vi "Save-As-Default (SubVI).vi"(0 "Current VI's Path":path, 1 "Load Settings":bool, 9 "Save Settings":bool, 12 "Save and Exit":bool) -> (4 "appended path":path, 8 "Save as Default Error":errorcluster, 15 "Application:Kind":T1(ring))   [LabVIEW 2012]
panel:
  # "Save As Defaults (SubVI) - Created by Blake Otting - October 2007"
  # "Last Updated 7/21/09"
  # "Connect As Shown \nin Main Program VI"
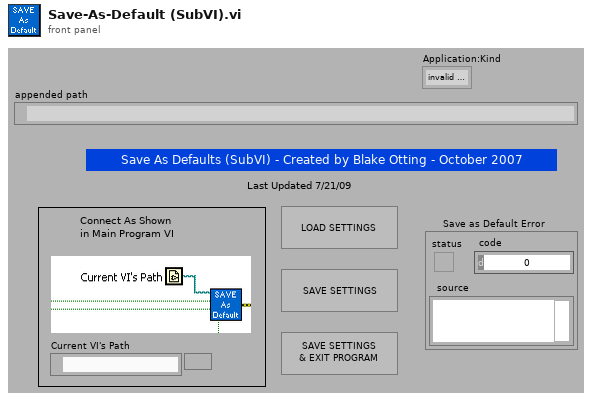
[diagram p1: front panel]
types:
  T1 = enum32{"invalid app kind", "Development System", "Run Time System", "Student Edition", "Embedded LabVIEW", "Evaluation", "Custom"}
  T2 = enum16{"open", "replace", "create", "open or create", "replace or create", "replace or create with confirmation"}
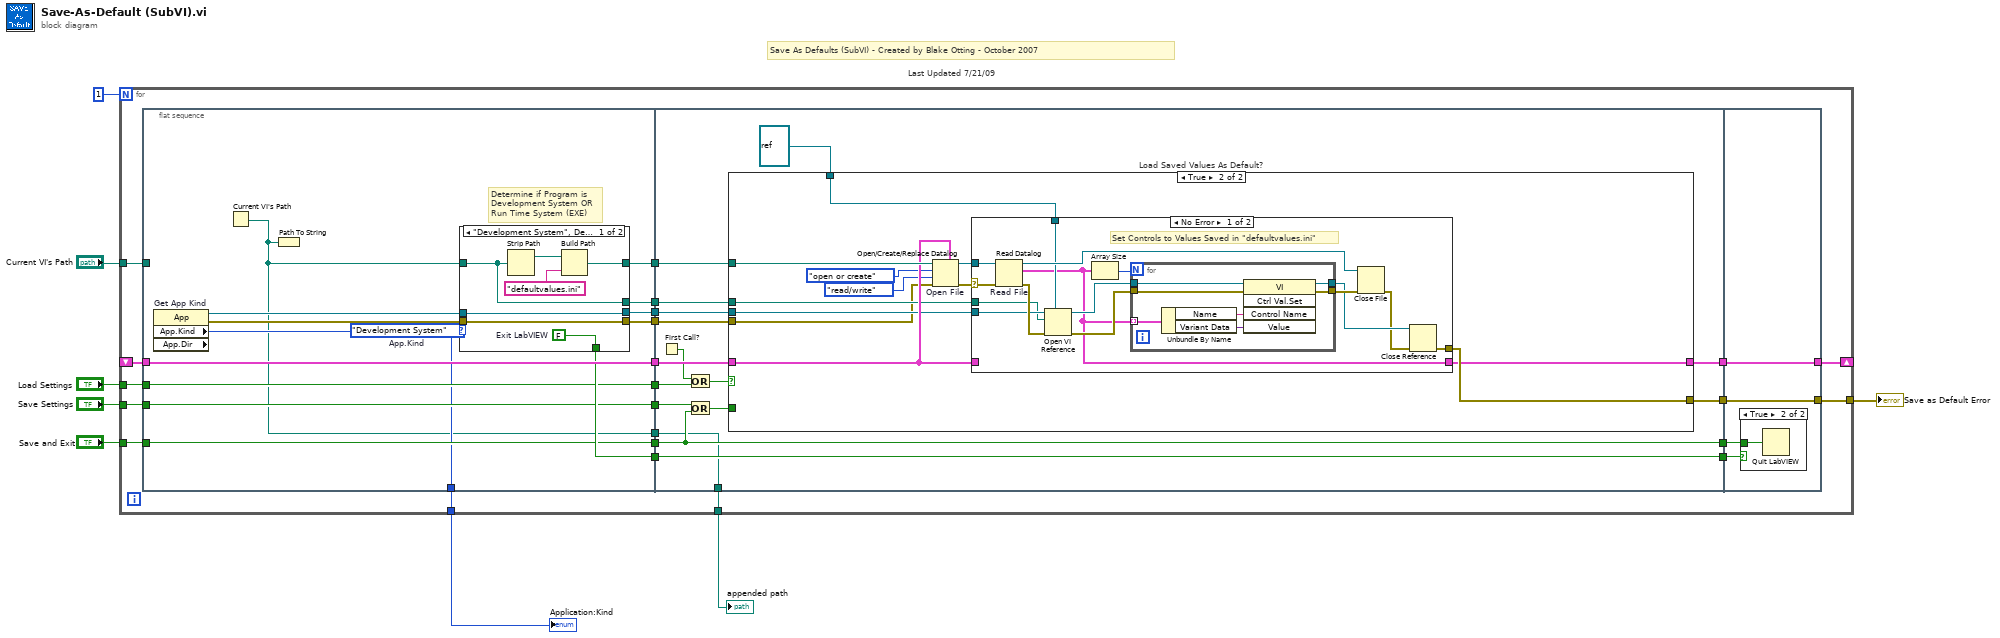
[diagram p0: block diagram]
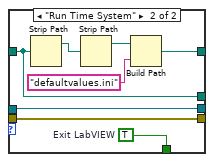
[diagram p2: hidden frame]
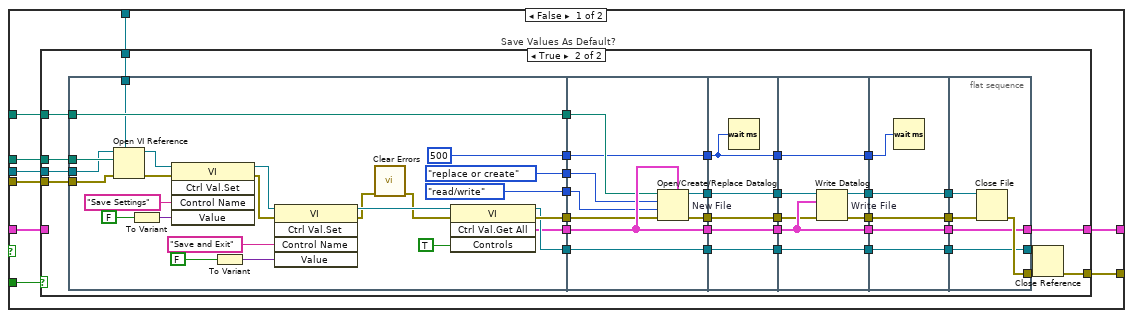
[diagram p3: hidden frame]
diagram:
  # "Last Updated 7/21/09"
  # "Save As Defaults (SubVI) - Created by Blake Otting - October 2007"
  n1 = for {
    N: 1 -> [_]
    tunnel: "Current VI's Path" -> [w30]
    shift-right: [w31] -> _
    shift-left: _ -> [w29]
    tunnel: [w28] -> w3
    tunnel: "Save and Exit" -> [w14]
    tunnel: "Load Settings" -> [w12]
    tunnel: "Save Settings" -> [w16]
    tunnel: [w11] -> w2
    tunnel: [w10] -> w1
    n2 = flat-sequence {
      tunnel: w30 -> [_]
      tunnel: w29 -> [w45]
      tunnel: [w45] -> w24
      tunnel: [w42] -> w23
      tunnel: [w41] -> w22
      tunnel: [w40] -> w21
      tunnel: [w39] -> w20
      tunnel: [w38] -> w19
      tunnel: [w37] -> w17
      tunnel: w16 -> [w37]
      tunnel: [w36] -> w15
      tunnel: w14 -> [w36]
      tunnel: [w35] -> w13
      tunnel: w12 -> [w35]
      tunnel: [w34] -> w11
      tunnel: [w32] -> w9
      tunnel: [w75] -> w27
      tunnel: [w68] -> w26
      tunnel: [w71] -> w25
      tunnel: w24 -> [w76]
      tunnel: w23 -> [w61]
      tunnel: w22 -> [w69]
      tunnel: w21 -> [w68]
      tunnel: w20 -> [w67]
      tunnel: w19 -> [w66]
      tunnel: [w65] -> w18
      tunnel: w17 -> [w64]
      tunnel: w15 -> [w65]
      tunnel: w13 -> [w63]
      tunnel: [w62] -> w10
      tunnel: w9 -> [w62]
      tunnel: [w217] -> w28
      tunnel: [w218] -> w31
      tunnel: w27 -> [w218]
      tunnel: w26 -> [w216]
      tunnel: w25 -> [w217]
      tunnel: w18 -> [w215]
      frame #0 {
        w33 = T1."Development System"  # App.Kind
        # "Determine if Program is\nDevelopment System OR\nRun Time System (EXE)"
        n3 = property on="Get App Kind" class="App" props=["App.Kind", "App.Dir"]() -> (reference out=w44:refnum<vi>, error out=w43:errorcluster, "App.Kind"=w34:T1)  [unwired: 2 in, 1 out]
        n4 = Current VI's Path() -> (path=w32:path)
        n5 = Path To String(path=w32) -> ()  [unwired: 1 out]
        n6 = case shown="\"Development System\", Default" w33 {
          tunnel: w43 -> [w52 w60]
          tunnel: [w52 w60] -> w41
          tunnel: w32 -> [w47 w54]
          tunnel: [w50 w56] -> w42
          tunnel: w44 -> [w48 w55]
          tunnel: [w48 w55] -> w38
          tunnel: [w47 w54] -> w39
          tunnel: [w46 w53] -> w40
          frame "Development System", Default {
            w46 = FALSE  # Exit LabVIEW
            n7 = Strip Path(path=w47) -> (stripped path=w49:path)  [unwired: 1 out]
            n8 = Build Path(base path=w49, name or relative path="defaultvalues.ini") -> (appended path=w50:path)
          }
          frame "Run Time System" {
            w53 = TRUE  # Exit LabVIEW
            n9 = Strip Path(path=w54) -> (stripped path=w57:path)  [unwired: 1 out]
            n10 = Strip Path(path=w57) -> (stripped path=w59:path)  [unwired: 1 out]
            n11 = Build Path(base path=w59, name or relative path="defaultvalues.ini") -> (appended path=w56:path)
          }
        }
      }
      frame #1 {
        n12 = First Call?() -> (First Call?: T/F=w70:bool)
        n13 = Or(x=w70, y=w63) -> (x .or. y?=w73:bool)
        n14 = Or(x=w64, y=w65) -> (x .or. y?=w72:bool)
        n15 = case "Load Saved Values As Default?" shown="True" w73 {
          tunnel: w69 -> [w85 w183]
          tunnel: [w84 w190] -> w71
          tunnel: w61 -> [w83 w188]
          tunnel: w72 -> [w82 _]
          tunnel: w76 -> [w81 w187]
          tunnel: [w77 w189] -> w75
          tunnel: w67 -> [w80 w184]
          tunnel: w66 -> [w79 w186]
          tunnel: refnum<vi> refnum ("Application Reference Input 2") -> [w78 w185]
          frame False {
            n16 = case "Save Values As Default?" shown="True" w82 {
              tunnel: w85 -> [w87 w88]
              tunnel: [w87 w122] -> w84
              tunnel: w83 -> [_ w121]
              tunnel: [w86 w120] -> w77
              tunnel: w81 -> [w86 _]
              tunnel: w80 -> [_ w90]
              tunnel: w79 -> [_ w89]
              tunnel: w78 -> [_ w91]
              frame False {
              }
              frame True {
                n17 = flat-sequence {
                  tunnel: w121 -> [w147]
                  tunnel: [w128] -> w100
                  tunnel: [enum16{"read/write", "read-only", "write-only"}."read/write" ("access (0:read/write)")] -> w99
                  tunnel: [T2."replace or create" ("operation (0:open)")] -> w98
                  tunnel: [w126] -> w97
                  tunnel: [w147] -> w96
                  tunnel: [w127] -> w95
                  tunnel: [u32 500 ("milliseconds to wait")] -> w94
                  tunnel: w91 -> [w131]
                  tunnel: w90 -> [w130]
                  tunnel: w89 -> [w129]
                  tunnel: w88 -> [w125]
                  tunnel: [w152] -> w119
                  tunnel: [w151] -> w117
                  tunnel: [w156] -> w115
                  tunnel: [w149] -> w113
                  tunnel: [w148] -> w101
                  tunnel: w100 -> [w155]
                  tunnel: w99 -> [w154]
                  tunnel: w98 -> [w153]
                  tunnel: w97 -> [w156]
                  tunnel: w96 -> [w150]
                  tunnel: w95 -> [w149]
                  tunnel: w94 -> [w148]
                  tunnel: w119 -> [w161]
                  tunnel: [w161] -> w118
                  tunnel: w117 -> [w160]
                  tunnel: [w160] -> w116
                  tunnel: w115 -> [w159]
                  tunnel: [w159] -> w114
                  tunnel: w113 -> [w158]
                  tunnel: [w158] -> w112
                  tunnel: w101 -> [w157]
                  tunnel: [w157] -> w92
                  tunnel: w118 -> [w166]
                  tunnel: w116 -> [w168]
                  tunnel: w114 -> [w167]
                  tunnel: [w167] -> w111
                  tunnel: w112 -> [w165]
                  tunnel: [w165] -> w109
                  tunnel: [w164] -> w107
                  tunnel: [w163] -> w105
                  tunnel: [w162] -> w93
                  tunnel: w92 -> [w162]
                  tunnel: w111 -> [w173]
                  tunnel: [w173] -> w110
                  tunnel: w109 -> [w172]
                  tunnel: [w172] -> w108
                  tunnel: w107 -> [w171]
                  tunnel: [w171] -> w106
                  tunnel: w105 -> [w170]
                  tunnel: [w170] -> w104
                  tunnel: w93 -> [w169]
                  tunnel: [w177] -> w120
                  tunnel: w110 -> [w177]
                  tunnel: [w176] -> w102
                  tunnel: w108 -> [w176]
                  tunnel: w106 -> [w175]
                  tunnel: w104 -> [w174]
                  tunnel: [w178] -> w103
                  frame #0 {
                    n18 = Open VI Reference(type specifier VI Refnum (for type only)=w131, application reference (local)=w129, vi path=w130, error in (no error)=w125) -> (vi reference=w139:refnum<vi>, error out=w140:errorcluster)  [unwired: 2 out]
                    n19 = To Variant(anything=FALSE ("Controls")) -> (Variant=w138:variant)
                    n20 = invoke class="VI" method="Ctrl Val.Set"(reference=w139, error in=w140, "Control Name"="Save Settings", "Value"=w138) -> (reference out=w143:refnum<vi>, error out=w144:errorcluster)  [unwired: 1 in, 3 out]
                    n21 = To Variant(anything=FALSE ("Controls")) -> (Variant=w141:variant)
                    n22 = invoke class="VI" method="Ctrl Val.Set"(reference=w143, error in=w144, "Control Name"="Save and Exit", "Value"=w141) -> (reference out=w146:refnum<vi>, error out=w124:errorcluster)  [unwired: 1 in, 3 out]
                    n23 = call <vilib>:"Clear Errors.vi"("error in (no error)"=w124) -> ("error out"=w123:errorcluster)  [unwired: 6 out]
                    n24 = invoke class="VI" method="Ctrl Val.Get All"(reference=w146, error in=w123, "Controls"=TRUE) -> (reference out=w127:refnum<vi>, error out=w128:errorcluster, "Get All Control Values Variant"=w126:cluster{"Name":string, "Variant Data":variant}[])  [unwired: 1 in, 1 out]
                  }
                  frame #1 {
                    n25 = Open/Create/Replace Datalog "New File"(5:w156, 8:w155, 9:w154, 10:w153, 11:w150) -> (0:w152:errorcluster, 3:w151:refnum<k1>)  [unwired: 2 out]
                  }
                  frame #2 {
                    n26 = Wait (ms)(milliseconds to wait=w157) -> ()  [unwired: 1 out]
                  }
                  frame #3 {
                    n27 = Write Datalog "Write File"(4:w166, 6:w167, 7:w168) -> (0:w164:errorcluster, 3:w163:refnum<k1>)
                  }
                  frame #4 {
                    n28 = Wait (ms)(milliseconds to wait=w169) -> ()  [unwired: 1 out]
                  }
                  frame #5 {
                    n29 = Close File(refnum=w174, error in=w175) -> (error out=w178:errorcluster)  [unwired: 1 out]
                  }
                }
                n30 = Close Reference(reference=w102, error in (no error)=w103) -> (error out=w122:errorcluster)
              }
            }
          }
          frame True {
            n31 = Open/Create/Replace Datalog "Open File"(5:w187, 8:w183, 9:enum16{"read/write", "read-only", "write-only"}."read/write" ("access (0:read/write)"), 10:T2."open or create" ("operation (0:open)"), 11:w188) -> (0:w182:errorcluster, 3:w181:refnum<k1>)  [unwired: 2 out]
            n32 = case shown="No Error" w182 {
              selector: w182 -> [w199 w213]
              tunnel: [w203 w213] -> w190
              tunnel: w187 -> [_ w214]
              tunnel: [w191 w214] -> w189
              tunnel: w181 -> [w200 _]
              tunnel: w186 -> [w196 _]
              tunnel: w185 -> [w195 _]
              tunnel: w184 -> [w194 _]
              frame No Error {
                # "Set Controls to Values Saved in \"defaultvalues.ini\""
                n33 = Read Datalog "Read File"(4:w199, 7:w200) -> (0:w197:errorcluster, 2:w191:cluster{"Name":string, "Variant Data":variant}[], 3:w205:refnum<k1>)  [unwired: 1 out]
                n34 = Open VI Reference(type specifier VI Refnum (for type only)=w195, application reference (local)=w196, vi path=w194, error in (no error)=w197) -> (vi reference=w198:refnum<vi>, error out=w193:errorcluster)  [unwired: 2 out]
                n35 = Array Size(array=w191) -> (size(s)=w192:i32)
                n36 = for {
                  N: w192 -> [_]
                  tunnel: w191 -> [w208] mode=indexing
                  tunnel: w193 -> [w210]
                  tunnel: [w211] -> w204
                  tunnel: w198 -> [w209]
                  tunnel: [w206] -> w202
                  n37 = Unbundle By Name(w208) -> ("Name"=w207:string, "Variant Data"=w212:variant)
                  n38 = invoke class="VI" method="Ctrl Val.Set"(reference=w209, error in=w210, "Control Name"=w207, "Value"=w212) -> (reference out=w206:refnum<vi>, error out=w211:errorcluster)  [unwired: 1 in, 3 out]
                }
                n39 = Close File(refnum=w205, error in=w204) -> (error out=w201:errorcluster)  [unwired: 1 out]
                n40 = Close Reference(reference=w202, error in (no error)=w201) -> (error out=w203:errorcluster)
              }
              frame Error {
                # "\"defaultvalues.ini\" Not Found"
              }
            }
          }
        }
      }
      frame #2 {
        n41 = case shown="True" w216 {
          tunnel: w215 -> [_ w219]
          frame False {
          }
          frame True {
            n42 = Quit LabVIEW(quit? (T)=w219) -> ()
          }
        }
      }
    }
  }
  "Save as Default Error" <- w3
  "Application:Kind" <- w2
  "appended path" <- w1
